vi "Read Command.vi"(8 "error in (no error)":errorcluster, 11 "DriveData in":refnum<class "DriveData.lvclass">) -> (0 "error out":errorcluster, 2 "Command":T1, 3 "DriveData out":refnum<class "DriveData.lvclass">)   [LabVIEW 2017, in "DriveData.lvclass"]
uses:
  DriveData.lvclass
  Command.ctl
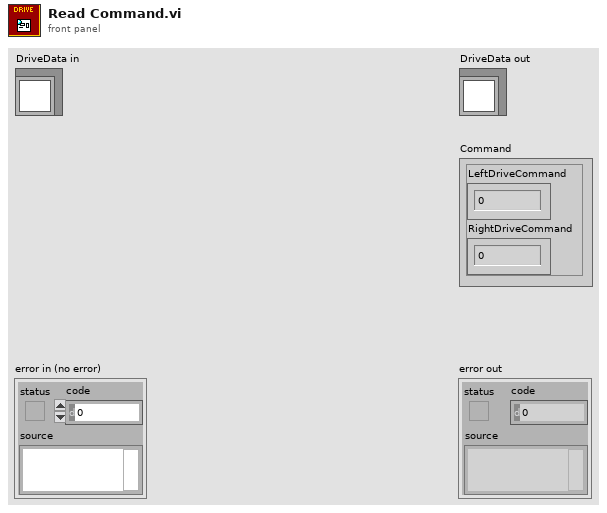
[diagram p1: front panel]
types:
  T1 = typedef "DriveData.lvclass/Command.ctl" = cluster{"LeftDriveCommand":dbl, "RightDriveCommand":dbl}
  T2 = cluster{"LeftDriveCommand":dbl, "RightDriveCommand":dbl}
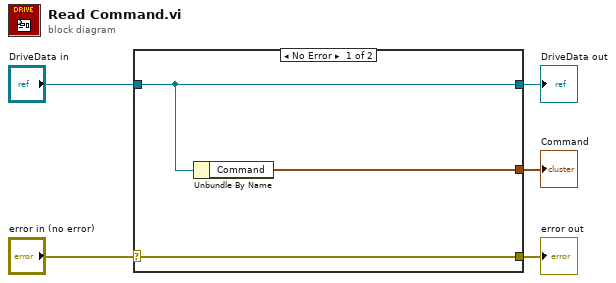
[diagram p0: block diagram]
diagram:
  n1 = case shown="No Error" "error in (no error)" {
    selector: "error in (no error)" -> [w8 w9]
    tunnel: [w8 w9] -> w4
    tunnel: [w7 w10] -> w2
    tunnel: "DriveData in" -> [w7 w10]
    tunnel: [w6 _] -> w1
    frame No Error {
      n2 = Unbundle By Name(w7) -> ("Command"=w6:T2)
    }
    frame Error {
    }
  }
  "error out" <- w4
  "DriveData out" <- w2
  "Command" <- w1
